vi "Test Fluke.vi"() -> ()   [LabVIEW 2019]
uses:
  Fluke Configuration.ctl
  Fluke 1586A Driver.lvclass
  C:/GitHub/NHMFL_Core/Libraries/Instruments/VISA Instrument/VISA Instrument.lvclass
  C:/GitHub/NHMFL_Core/Libraries/Instruments/Instrument Driver/Instrument Driver.lvclass
  VISA Instrument/VISA Instrument.lvclass/VISA Instrument.ctl
  VISA Instrument/Write VISA resource.vi
  Instrument Driver/Write User configuration.vi
  GPIB/VISA  Send Receive.vi
panel:
  in  "Configuration":T1={"Channels"="201:203"}
  out "Measure cycle":i32
  in  "milliseconds to wait at init":u32=100
  in  "milliseconds to wait":u32=100
  in  "Stop Button":bool
  out "Status loop index":i32
  out "Data ready":bool
  in  "Receive count":i32=256
  in  "Read Delay, ms":u32=10000
  out "data string out":string
  in  "data string in":string="FUNC \"FRES\",(@201:204);ROUT:SCAN (@201:204);READ?"
  out "Array - Numeric":dbl[](array[numeric])=[109.724]
  out "IDN":string="FLUKE,1586A,47035007,1.04+1.02+20130618\n"
  in  "VISA resource name":refnum<visa-resource-name>="TCPIP0::192.168.1.100::3490::SOCKET"
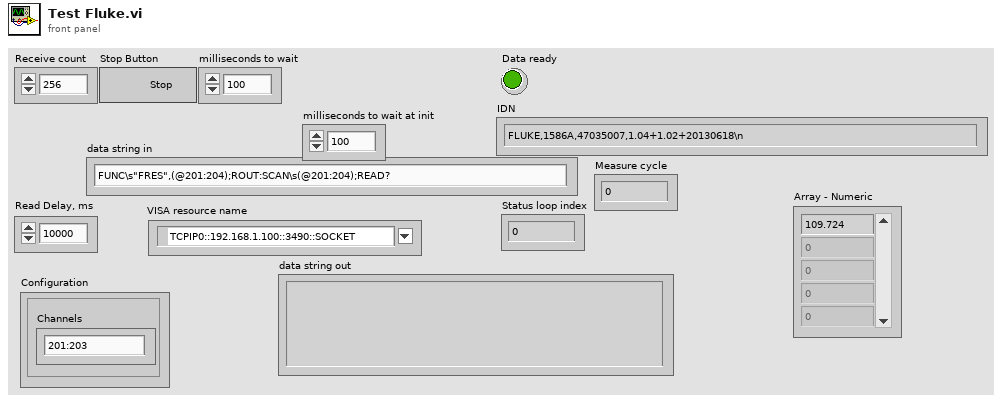
[diagram p1: front panel]
types:
  T1 = typedef "Fluke Configuration.ctl" = cluster{"Channels":string}
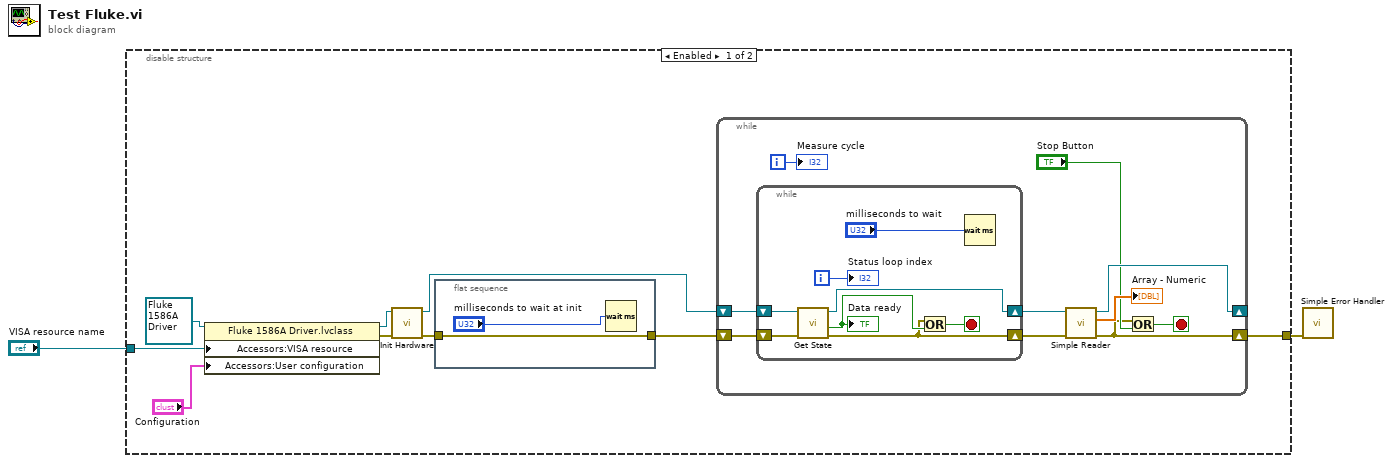
[diagram p0: block diagram]
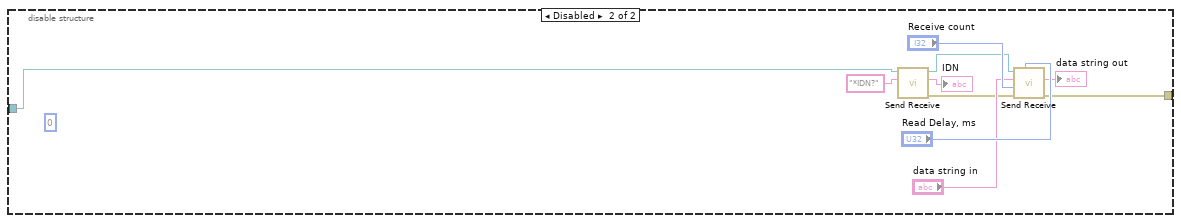
[diagram p2: hidden frame]
diagram:
  n1 = disable-structure shown="Enabled" {
    disable-tunnel: [w9 w33] -> w1
    disable-tunnel: "VISA resource name" -> [w8 w32]
    frame Enabled {
      n2 = property class="Fluke 1586A Driver.lvclass"(reference=refnum<class "Fluke 1586A Driver.lvclass"> refnum ("Fluke 1586A Driver.lvclass"), "Accessors:VISA resource"=w8, "Accessors:User configuration"="Configuration") -> (reference out=w7:refnum<class "Fluke 1586A Driver.lvclass">, error out=w10:errorcluster)  [unwired: 1 in]
      n3 = call-dynamic "Init Hardware.vi"("error in (no error)"=w10, "Fluke 1586A Driver in"=w7) -> ("error out"=w6:errorcluster, "Fluke 1586A Driver out"=w5:refnum<class "Fluke 1586A Driver.lvclass">)  [unwired: 8 in]
      n4 = flat-sequence {
        tunnel: [w13] -> w3
        tunnel: w6 -> [w13]
        frame #0 {
          n5 = Wait (ms)(milliseconds to wait="milliseconds to wait at init") -> ()  [unwired: 1 out]
        }
      }
      n6 = while {
        shift-right: [w15] -> w9
        shift-left: w3 -> [w22]
        shift-right: [w18] -> _
        shift-left: w5 -> [w20]
        i -> [w14]
        stop <- w16 stop-if-true
        n7 = while {
          shift-right: [w25] -> w21
          shift-left: w22 -> [w31]
          shift-right: [w29] -> w19
          shift-left: w20 -> [w30]
          i -> [w27]
          stop <- w26 stop-if-true
          n8 = call-dynamic "Get State.vi"("error in (no error)"=w31, "Fluke 1586A Driver in"=w30) -> ("error out"=w25:errorcluster, "Data ready"=w28:bool, "Fluke 1586A Driver out"=w29:refnum<class "Fluke 1586A Driver.lvclass">)  [unwired: 4 in, 3 out]
          "Data ready" <- w28
          n9 = Or(x=w25, y=w28) -> (x .or. y?=w26:bool)
          n10 = Wait (ms)(milliseconds to wait="milliseconds to wait") -> ()  [unwired: 1 out]
          "Status loop index" <- w27
        }
        n11 = call-dynamic "Simple Reader.vi"("error in (no error)"=w21, "Fluke 1586A Driver in"=w19) -> ("error out"=w15:errorcluster, "Signals"=→"Array - Numeric":dbl[], "Fluke 1586A Driver out"=w18:refnum<class "Fluke 1586A Driver.lvclass">)  [unwired: 7 in]
        n12 = Or(x=w15, y="Stop Button") -> (x .or. y?=w16:bool)
        "Measure cycle" <- w14
      }
    }
    frame Disabled {
      (unwired) 0 ("Receive count")
      n13 = call-poly "Send Receive.vi"("data string in"="*IDN?", "VISA Resource Name"=w32) -> ("error out"=w37:errorcluster, "data string out"=→"IDN":string, "VISA Resource Name Out"=w36:refnum<visa-resource-name>)  [unwired: 7 in]
      n14 = call-poly "Send Receive.vi"("Read Delay, ms"="Read Delay, ms", "error in (no error)"=w37, "Receive count"="Receive count", "data string in"="data string in", "VISA Resource Name"=w36) -> ("error out"=w33:errorcluster, "data string out"=→"data string out":string)  [unwired: 4 in, 1 out]
    }
  }
  n15 = call <vilib>:"Simple Error Handler.vi"("error in (no error)"=w1) -> ()  [unwired: 4 in, 5 out]
